vi "c ctre phoenixpro serialize bool no malloc.vi"(7 "max_len":u32, 8 "error in (no error)":errorcluster, 9 "str":string, 10 "value":bool, 11 "spn":i32) -> (0 "error out":errorcluster, 1 "str out":string, 3 "function return":i32)   [LabVIEW 2020, in "CTRE_PhoenixTools.lvlib"]
doc: "CTREXPORT int c_ctre_phoenixpro_serialize_bool_no_malloc(int spn, bool value, char *str, uint32_t max_len);"
uses:
  CTRE_PhoenixTools.lvlib
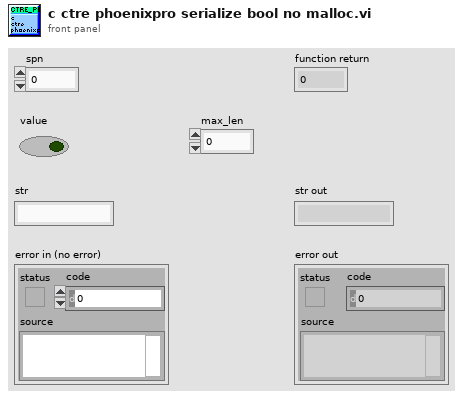
[diagram p1: front panel]
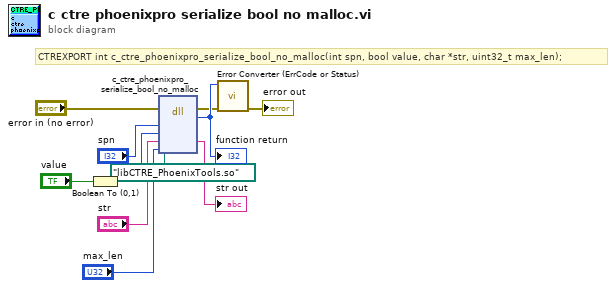
[diagram p0: block diagram]
diagram:
  # "CTREXPORT int c_ctre_phoenixpro_serialize_bool_no_malloc(int spn, bool value, char *str, uint32_t max_len);"
  n1 = Boolean To (0,1)(Boolean="value") -> (0, 1=w8:i16)
  n2 = dll-call lib="?" fn="c_ctre_phoenixpro_serialize_bool_no_malloc"(path in=path "libCTRE_PhoenixTools.so", error in="error in (no error)", "spn"="spn", "value"=w8, "str"="str", "max_len"="max_len") -> (error out=w3:errorcluster, w11:i32, "str"=→"str out":string)  [unwired: 4 in, 1 out]
  "function return" <- w11
  n3 = call "Error Converter (ErrCode or Status).vi"("error in (no error)"=w3, "error code"=w11) -> ("error out"=→"error out":errorcluster)  [unwired: 9 in]
